vi "OnePointSub.vi"(3 "cluster":T1) -> (0 "TextArray":string[](array[string]), 1 "Array":dbl[](array[numeric]))   [LabVIEW 2017]
panel:
  out "Numeric 3":i32
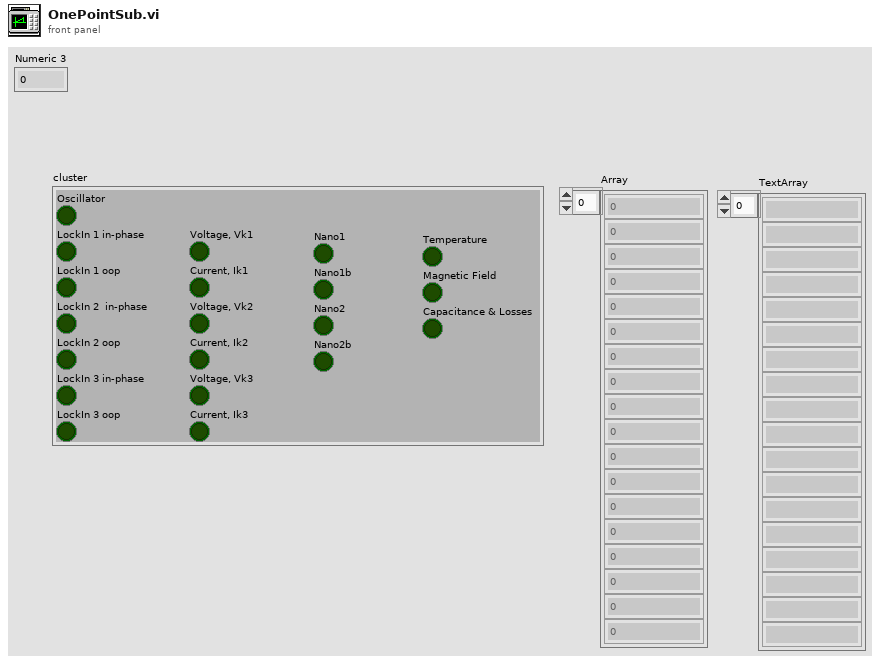
[diagram p1: front panel]
types:
  T1 = cluster{"Oscillator":bool, "LockIn 1 in-phase":bool, "LockIn 1 oop ":bool, "LockIn 2  in-phase":bool, "LockIn 2 oop":bool, "LockIn 3 in-phase":bool, "LockIn 3 oop":bool, "Voltage, Vk1":bool, "Current, Ik1":bool, "Voltage, Vk2":bool, "Current, Ik2":bool, "Voltage, Vk3":bool, "Current, Ik3":bool, "Nano1":bool, "Nano1b":bool, "Nano2":bool, "Nano2b":bool, "Temperature":bool, "Magnetic Field":bool, "Capacitance & Losses":bool}
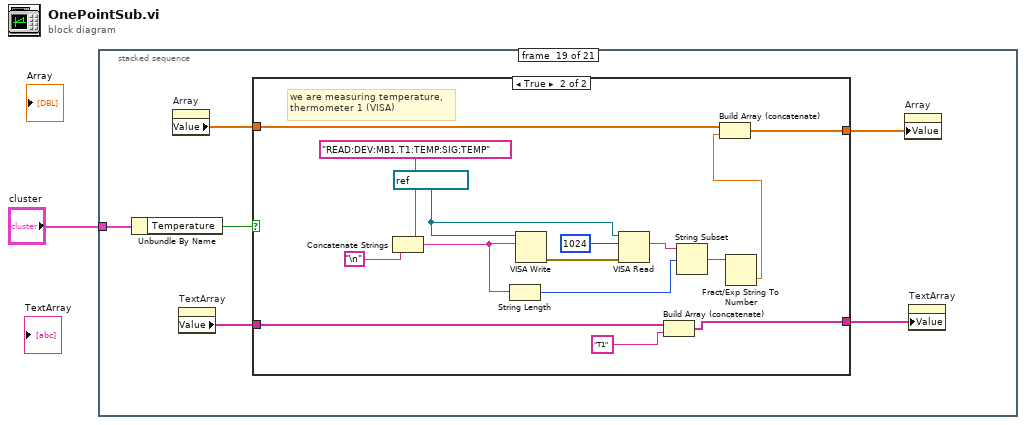
[diagram p0: block diagram]
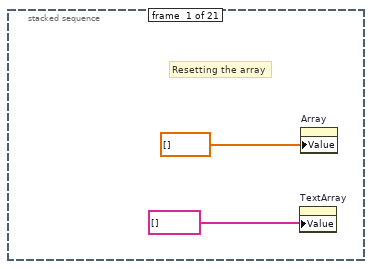
[diagram p2: hidden frame]
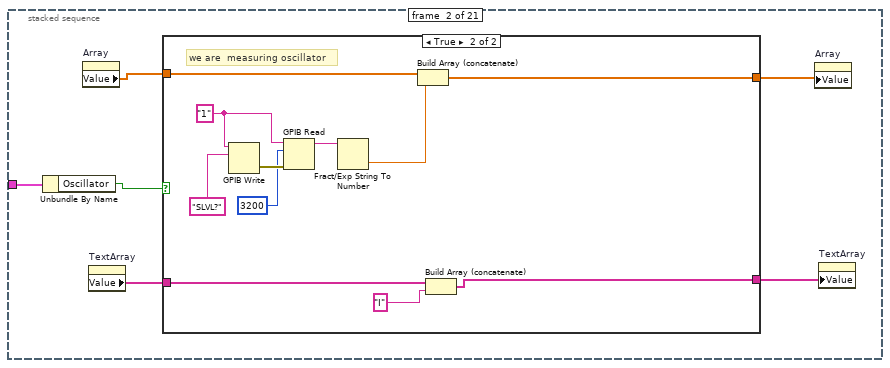
[diagram p3: hidden frame]
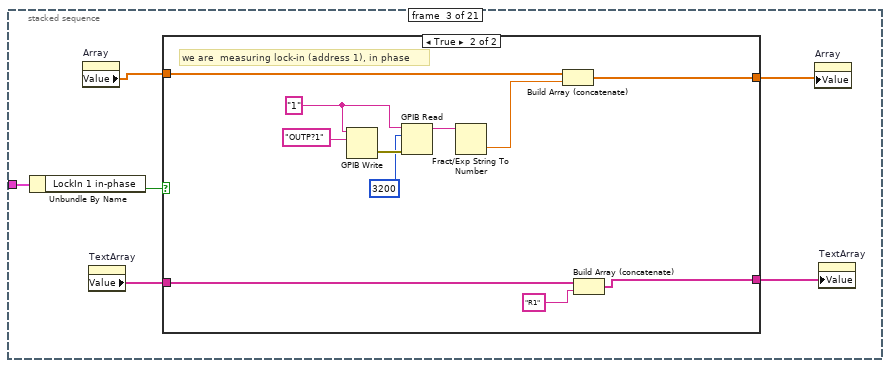
[diagram p5: hidden frame]
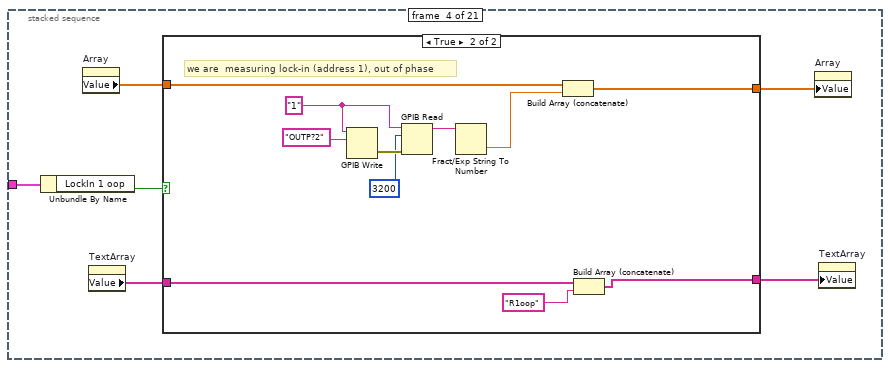
[diagram p7: hidden frame]
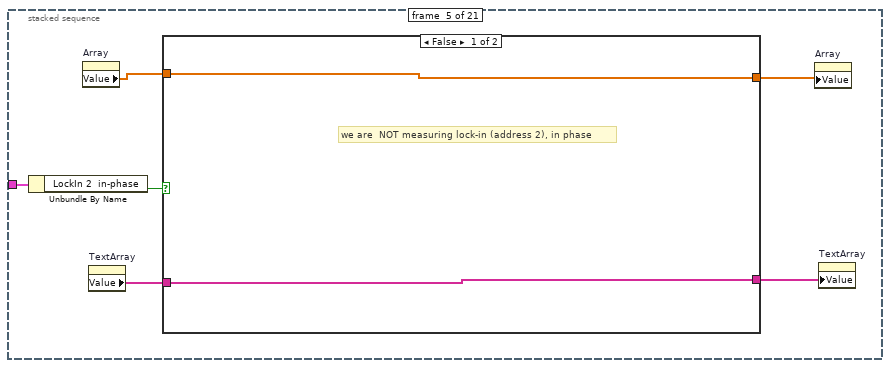
[diagram p9: hidden frame]
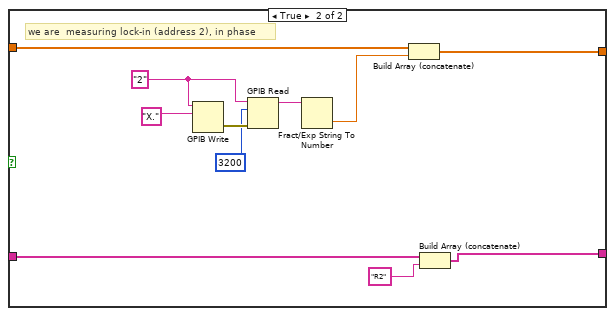
[diagram p10: hidden frame]
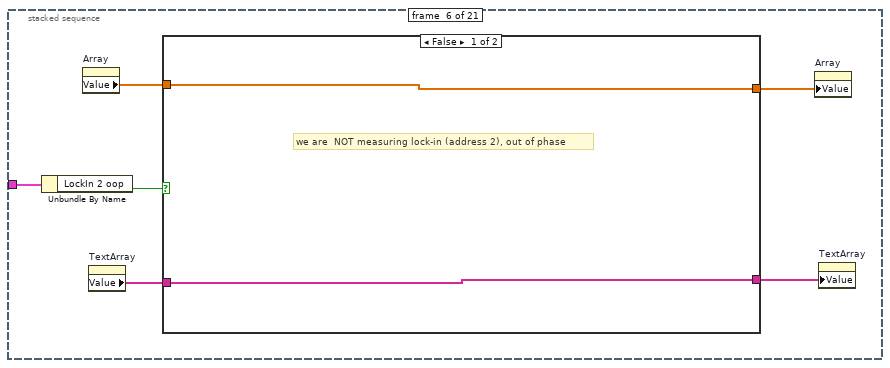
[diagram p11: hidden frame]
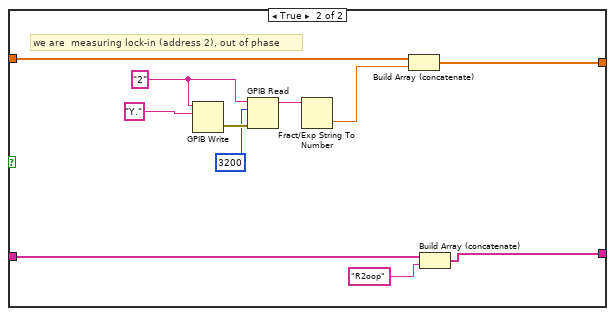
[diagram p12: hidden frame]
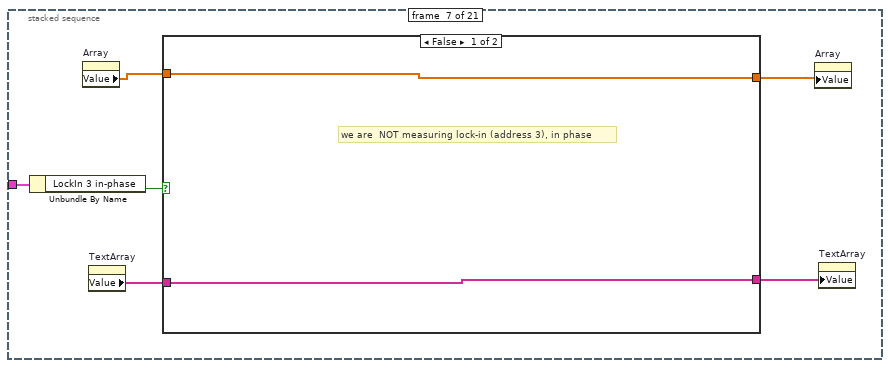
[diagram p13: hidden frame]
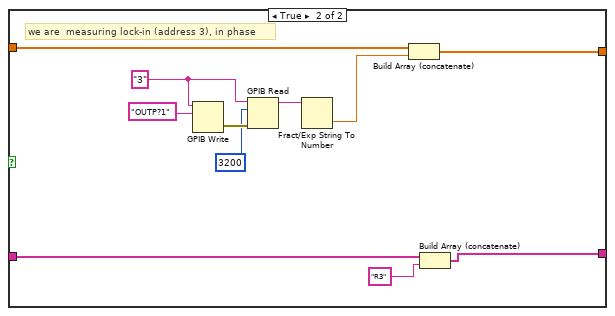
[diagram p14: hidden frame]
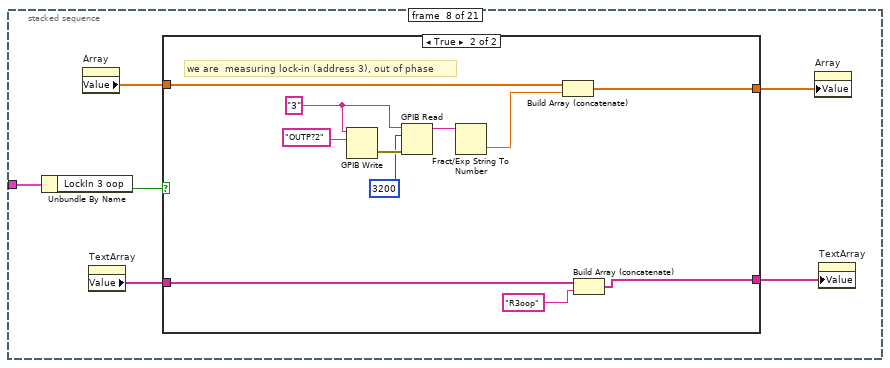
[diagram p15: hidden frame]
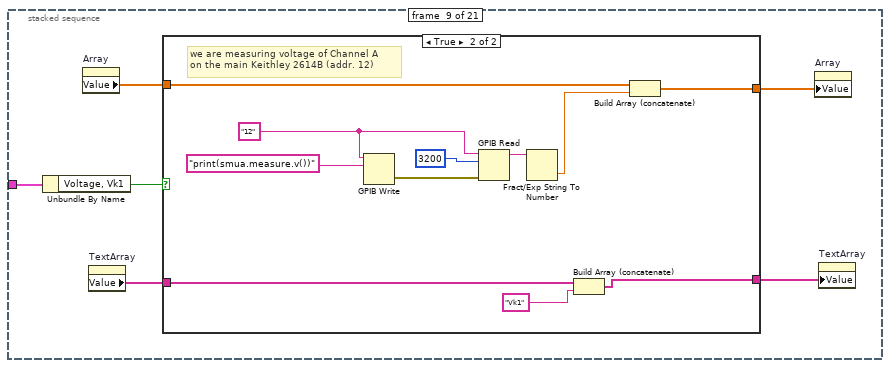
[diagram p17: hidden frame]
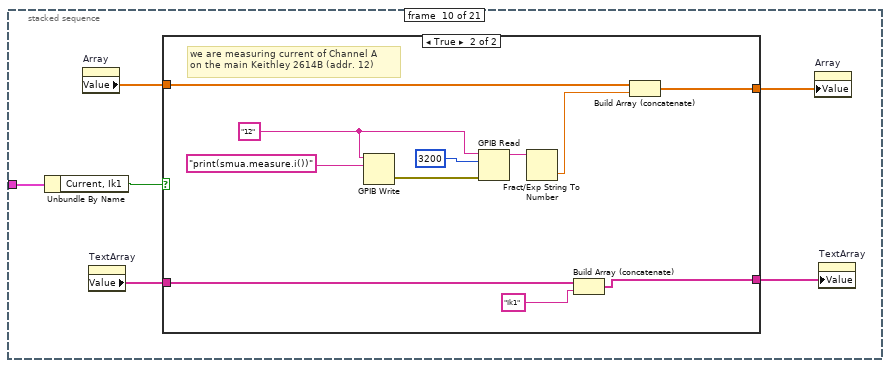
[diagram p19: hidden frame]
diagram:
  n1 = stacked-sequence {
    tunnel: "cluster" -> [_ w9 w28 w47 w66 w85 w104 w123 w142 w161 w180 w199 w218 w237 w256 w275 w298 w317 w340 w363 w386]
    frame #0 {
      # "Resetting the array"
      n2 = property on="TextArray" class="Arr (strict)"("Value"=string[] []) -> ()  [unwired: 2 in, 2 out]
      n3 = property on="Array" class="Arr (strict)"("Value"=dbl[] []) -> ()  [unwired: 2 in, 2 out]
    }
    frame #1 {
      n4 = Unbundle By Name(w9) -> ("Oscillator"=w6:bool)
      n5 = property on="Array" class="Arr (strict)"() -> ("Value"=w8:dbl[])  [unwired: 2 in, 2 out]
      n6 = property on="TextArray" class="Arr (strict)"() -> ("Value"=w5:string[])  [unwired: 2 in, 2 out]
      n7 = case shown="True" w6 {
        tunnel: w8 -> [w11 w22]
        tunnel: [w11 w21] -> w7
        tunnel: w5 -> [w10 w14]
        tunnel: [w10 w13] -> w4
        frame False {
          # "we are not measuring oscillator from\nlock-in (address 1)"
        }
        frame True {
          w18 = "1"
          # "we are  measuring oscillator"
          n8 = GPIB Write(0:w18, 1:"SLVL?") -> (6:w19:errorcluster)  [unwired: 3 in, 1 out]
          n9 = GPIB Read(0:w18, 1:3200, 3:w19) -> (5:w16:string)  [unwired: 2 in, 2 out]
          n10 = Fract/Exp String To Number(string=w16) -> (number=w15:dbl)  [unwired: 3 in, 1 out]
          n11 = Build Array (concatenate)(w22, w15) -> (w21:dbl[])
          n12 = Build Array (concatenate)(w14, "I") -> (w13:string[])
        }
      }
      n13 = property on="Array" class="Arr (strict)"("Value"=w7) -> ()  [unwired: 2 in, 2 out]
      n14 = property on="TextArray" class="Arr (strict)"("Value"=w4) -> ()  [unwired: 2 in, 2 out]
    }
    frame #2 {
      n15 = Unbundle By Name(w28) -> ("LockIn 1 in-phase"=w25:bool)
      n16 = property on="Array" class="Arr (strict)"() -> ("Value"=w27:dbl[])  [unwired: 2 in, 2 out]
      n17 = property on="TextArray" class="Arr (strict)"() -> ("Value"=w24:string[])  [unwired: 2 in, 2 out]
      n18 = case shown="True" w25 {
        tunnel: w27 -> [w30 w41]
        tunnel: [w30 w40] -> w26
        tunnel: w24 -> [w29 w39]
        tunnel: [w29 w38] -> w23
        frame False {
          # "we are  NOT measuring lock-in (address 1), in phase"
        }
        frame True {
          w35 = "1"
          # "we are  measuring lock-in (address 1), in phase"
          n19 = GPIB Write(0:w35, 1:"OUTP?1") -> (6:w36:errorcluster)  [unwired: 3 in, 1 out]
          n20 = GPIB Read(0:w35, 1:3200, 3:w36) -> (5:w33:string)  [unwired: 2 in, 2 out]
          n21 = Fract/Exp String To Number(string=w33) -> (number=w31:dbl)  [unwired: 3 in, 1 out]
          n22 = Build Array (concatenate)(w41, w31) -> (w40:dbl[])
          n23 = Build Array (concatenate)(w39, "R1") -> (w38:string[])
        }
      }
      n24 = property on="Array" class="Arr (strict)"("Value"=w26) -> ()  [unwired: 2 in, 2 out]
      n25 = property on="TextArray" class="Arr (strict)"("Value"=w23) -> ()  [unwired: 2 in, 2 out]
    }
    frame #3 {
      n26 = Unbundle By Name(w47) -> ("LockIn 1 oop"=w44:bool)
      n27 = property on="Array" class="Arr (strict)"() -> ("Value"=w46:dbl[])  [unwired: 2 in, 2 out]
      n28 = property on="TextArray" class="Arr (strict)"() -> ("Value"=w43:string[])  [unwired: 2 in, 2 out]
      n29 = case shown="True" w44 {
        tunnel: w46 -> [w49 w60]
        tunnel: [w49 w59] -> w45
        tunnel: w43 -> [w48 w58]
        tunnel: [w48 w57] -> w42
        frame False {
          # "we are  NOT measuring lock-in (address 1), out of phase"
        }
        frame True {
          w54 = "1"
          # "we are  measuring lock-in (address 1), out of phase"
          n30 = GPIB Write(0:w54, 1:"OUTP?2") -> (6:w55:errorcluster)  [unwired: 3 in, 1 out]
          n31 = GPIB Read(0:w54, 1:3200, 3:w55) -> (5:w52:string)  [unwired: 2 in, 2 out]
          n32 = Fract/Exp String To Number(string=w52) -> (number=w50:dbl)  [unwired: 3 in, 1 out]
          n33 = Build Array (concatenate)(w60, w50) -> (w59:dbl[])
          n34 = Build Array (concatenate)(w58, "R1oop") -> (w57:string[])
        }
      }
      n35 = property on="Array" class="Arr (strict)"("Value"=w45) -> ()  [unwired: 2 in, 2 out]
      n36 = property on="TextArray" class="Arr (strict)"("Value"=w42) -> ()  [unwired: 2 in, 2 out]
    }
    frame #4 {
      n37 = Unbundle By Name(w66) -> ("LockIn 2  in-phase"=w63:bool)
      n38 = property on="Array" class="Arr (strict)"() -> ("Value"=w65:dbl[])  [unwired: 2 in, 2 out]
      n39 = property on="TextArray" class="Arr (strict)"() -> ("Value"=w62:string[])  [unwired: 2 in, 2 out]
      n40 = case shown="False" w63 {
        tunnel: w65 -> [w68 w79]
        tunnel: [w68 w78] -> w64
        tunnel: w62 -> [w67 w77]
        tunnel: [w67 w76] -> w61
        frame False {
          # "we are  NOT measuring lock-in (address 2), in phase"
        }
        frame True {
          w73 = "2"
          # "we are  measuring lock-in (address 2), in phase"
          n41 = GPIB Write(0:w73, 1:"X.") -> (6:w74:errorcluster)  [unwired: 3 in, 1 out]
          n42 = GPIB Read(0:w73, 1:3200, 3:w74) -> (5:w71:string)  [unwired: 2 in, 2 out]
          n43 = Fract/Exp String To Number(string=w71) -> (number=w70:dbl)  [unwired: 3 in, 1 out]
          n44 = Build Array (concatenate)(w79, w70) -> (w78:dbl[])
          n45 = Build Array (concatenate)(w77, "R2") -> (w76:string[])
        }
      }
      n46 = property on="Array" class="Arr (strict)"("Value"=w64) -> ()  [unwired: 2 in, 2 out]
      n47 = property on="TextArray" class="Arr (strict)"("Value"=w61) -> ()  [unwired: 2 in, 2 out]
    }
    frame #5 {
      n48 = Unbundle By Name(w85) -> ("LockIn 2 oop"=w82:bool)
      n49 = property on="Array" class="Arr (strict)"() -> ("Value"=w84:dbl[])  [unwired: 2 in, 2 out]
      n50 = property on="TextArray" class="Arr (strict)"() -> ("Value"=w81:string[])  [unwired: 2 in, 2 out]
      n51 = case shown="False" w82 {
        tunnel: w84 -> [w87 w98]
        tunnel: [w87 w97] -> w83
        tunnel: w81 -> [w86 w96]
        tunnel: [w86 w95] -> w80
        frame False {
          # "we are  NOT measuring lock-in (address 2), out of phase"
        }
        frame True {
          w92 = "2"
          # "we are  measuring lock-in (address 2), out of phase"
          n52 = GPIB Write(0:w92, 1:"Y.") -> (6:w93:errorcluster)  [unwired: 3 in, 1 out]
          n53 = GPIB Read(0:w92, 1:3200, 3:w93) -> (5:w90:string)  [unwired: 2 in, 2 out]
          n54 = Fract/Exp String To Number(string=w90) -> (number=w88:dbl)  [unwired: 3 in, 1 out]
          n55 = Build Array (concatenate)(w98, w88) -> (w97:dbl[])
          n56 = Build Array (concatenate)(w96, "R2oop") -> (w95:string[])
        }
      }
      n57 = property on="Array" class="Arr (strict)"("Value"=w83) -> ()  [unwired: 2 in, 2 out]
      n58 = property on="TextArray" class="Arr (strict)"("Value"=w80) -> ()  [unwired: 2 in, 2 out]
    }
    frame #6 {
      n59 = Unbundle By Name(w104) -> ("LockIn 3 in-phase"=w101:bool)
      n60 = property on="Array" class="Arr (strict)"() -> ("Value"=w103:dbl[])  [unwired: 2 in, 2 out]
      n61 = property on="TextArray" class="Arr (strict)"() -> ("Value"=w100:string[])  [unwired: 2 in, 2 out]
      n62 = case shown="False" w101 {
        tunnel: w103 -> [w106 w117]
        tunnel: [w106 w116] -> w102
        tunnel: w100 -> [w105 w115]
        tunnel: [w105 w114] -> w99
        frame False {
          # "we are  NOT measuring lock-in (address 3), in phase"
        }
        frame True {
          w111 = "3"
          # "we are  measuring lock-in (address 3), in phase"
          n63 = GPIB Write(0:w111, 1:"OUTP?1") -> (6:w112:errorcluster)  [unwired: 3 in, 1 out]
          n64 = GPIB Read(0:w111, 1:3200, 3:w112) -> (5:w109:string)  [unwired: 2 in, 2 out]
          n65 = Fract/Exp String To Number(string=w109) -> (number=w107:dbl)  [unwired: 3 in, 1 out]
          n66 = Build Array (concatenate)(w117, w107) -> (w116:dbl[])
          n67 = Build Array (concatenate)(w115, "R3") -> (w114:string[])
        }
      }
      n68 = property on="Array" class="Arr (strict)"("Value"=w102) -> ()  [unwired: 2 in, 2 out]
      n69 = property on="TextArray" class="Arr (strict)"("Value"=w99) -> ()  [unwired: 2 in, 2 out]
    }
    frame #7 {
      n70 = Unbundle By Name(w123) -> ("LockIn 3 oop"=w120:bool)
      n71 = property on="Array" class="Arr (strict)"() -> ("Value"=w122:dbl[])  [unwired: 2 in, 2 out]
      n72 = property on="TextArray" class="Arr (strict)"() -> ("Value"=w119:string[])  [unwired: 2 in, 2 out]
      n73 = case shown="True" w120 {
        tunnel: w122 -> [w125 w136]
        tunnel: [w125 w135] -> w121
        tunnel: w119 -> [w124 w134]
        tunnel: [w124 w133] -> w118
        frame False {
          # "we are  NOT measuring lock-in (address 3), out of phase"
        }
        frame True {
          w130 = "3"
          # "we are  measuring lock-in (address 3), out of phase"
          n74 = GPIB Write(0:w130, 1:"OUTP?2") -> (6:w131:errorcluster)  [unwired: 3 in, 1 out]
          n75 = GPIB Read(0:w130, 1:3200, 3:w131) -> (5:w128:string)  [unwired: 2 in, 2 out]
          n76 = Fract/Exp String To Number(string=w128) -> (number=w126:dbl)  [unwired: 3 in, 1 out]
          n77 = Build Array (concatenate)(w136, w126) -> (w135:dbl[])
          n78 = Build Array (concatenate)(w134, "R3oop") -> (w133:string[])
        }
      }
      n79 = property on="Array" class="Arr (strict)"("Value"=w121) -> ()  [unwired: 2 in, 2 out]
      n80 = property on="TextArray" class="Arr (strict)"("Value"=w118) -> ()  [unwired: 2 in, 2 out]
    }
    frame #8 {
      n81 = Unbundle By Name(w142) -> ("Voltage, Vk1"=w139:bool)
      n82 = property on="Array" class="Arr (strict)"() -> ("Value"=w141:dbl[])  [unwired: 2 in, 2 out]
      n83 = property on="TextArray" class="Arr (strict)"() -> ("Value"=w138:string[])  [unwired: 2 in, 2 out]
      n84 = case shown="True" w139 {
        tunnel: w141 -> [w144 w155]
        tunnel: [w144 w154] -> w140
        tunnel: w138 -> [w143 w153]
        tunnel: [w143 w152] -> w137
        frame False {
          # "we are NOT measuring voltage of Channel A \non the main Keithley 2614B (addr. 12)"
        }
        frame True {
          w149 = "12"
          # "we are measuring voltage of Channel A \non the main Keithley 2614B (addr. 12)"
          n85 = GPIB Write(0:w149, 1:"print(smua.measure.v())") -> (6:w150:errorcluster)  [unwired: 3 in, 1 out]
          n86 = GPIB Read(0:w149, 1:3200, 3:w150) -> (5:w146:string)  [unwired: 2 in, 2 out]
          n87 = Fract/Exp String To Number(string=w146) -> (number=w145:dbl)  [unwired: 3 in, 1 out]
          n88 = Build Array (concatenate)(w153, "Vk1") -> (w152:string[])
          n89 = Build Array (concatenate)(w155, w145) -> (w154:dbl[])
        }
      }
      n90 = property on="Array" class="Arr (strict)"("Value"=w140) -> ()  [unwired: 2 in, 2 out]
      n91 = property on="TextArray" class="Arr (strict)"("Value"=w137) -> ()  [unwired: 2 in, 2 out]
    }
    frame #9 {
      n92 = Unbundle By Name(w161) -> ("Current, Ik1"=w158:bool)
      n93 = property on="Array" class="Arr (strict)"() -> ("Value"=w160:dbl[])  [unwired: 2 in, 2 out]
      n94 = property on="TextArray" class="Arr (strict)"() -> ("Value"=w157:string[])  [unwired: 2 in, 2 out]
      n95 = case shown="True" w158 {
        tunnel: w160 -> [w163 w174]
        tunnel: [w163 w173] -> w159
        tunnel: w157 -> [w162 w172]
        tunnel: [w162 w171] -> w156
        frame False {
          # "we are NOT measuring current of Channel A \non the main Keithley 2614B (addr. 12)"
        }
        frame True {
          w168 = "12"
          # "we are measuring current of Channel A \non the main Keithley 2614B (addr. 12)"
          n96 = GPIB Write(0:w168, 1:"print(smua.measure.i())") -> (6:w169:errorcluster)  [unwired: 3 in, 1 out]
          n97 = GPIB Read(0:w168, 1:3200, 3:w169) -> (5:w165:string)  [unwired: 2 in, 2 out]
          n98 = Fract/Exp String To Number(string=w165) -> (number=w164:dbl)  [unwired: 3 in, 1 out]
          n99 = Build Array (concatenate)(w172, "Ik1") -> (w171:string[])
          n100 = Build Array (concatenate)(w174, w164) -> (w173:dbl[])
        }
      }
      n101 = property on="Array" class="Arr (strict)"("Value"=w159) -> ()  [unwired: 2 in, 2 out]
      n102 = property on="TextArray" class="Arr (strict)"("Value"=w156) -> ()  [unwired: 2 in, 2 out]
    }
    frame #10 {
      n103 = Unbundle By Name(w180) -> ("Voltage, Vk2"=w177:bool)
      n104 = property on="Array" class="Arr (strict)"() -> ("Value"=w179:dbl[])  [unwired: 2 in, 2 out]
      n105 = property on="TextArray" class="Arr (strict)"() -> ("Value"=w176:string[])  [unwired: 2 in, 2 out]
      n106 = case shown="True" w177 {
        tunnel: w179 -> [w182 w193]
        tunnel: [w182 w192] -> w178
        tunnel: w176 -> [w181 w191]
        tunnel: [w181 w190] -> w175
        frame False {
          # "we are NOT measuring voltage of Channel B \non the main Keithley 2614B (addr. 12)"
        }
        frame True {
          w187 = "12"
          # "we are measuring voltage of Channel B \non the main Keithley 2614B (addr. 12)"
          n107 = GPIB Write(0:w187, 1:"print(smub.measure.v())") -> (6:w188:errorcluster)  [unwired: 3 in, 1 out]
          n108 = GPIB Read(0:w187, 1:3200, 3:w188) -> (5:w184:string)  [unwired: 2 in, 2 out]
          n109 = Fract/Exp String To Number(string=w184) -> (number=w183:dbl)  [unwired: 3 in, 1 out]
          n110 = Build Array (concatenate)(w191, "Vk2") -> (w190:string[])
          n111 = Build Array (concatenate)(w193, w183) -> (w192:dbl[])
        }
      }
      n112 = property on="Array" class="Arr (strict)"("Value"=w178) -> ()  [unwired: 2 in, 2 out]
      n113 = property on="TextArray" class="Arr (strict)"("Value"=w175) -> ()  [unwired: 2 in, 2 out]
    }
    frame #11 {
      n114 = Unbundle By Name(w199) -> ("Current, Ik2"=w196:bool)
      n115 = property on="Array" class="Arr (strict)"() -> ("Value"=w198:dbl[])  [unwired: 2 in, 2 out]
      n116 = property on="TextArray" class="Arr (strict)"() -> ("Value"=w195:string[])  [unwired: 2 in, 2 out]
      n117 = case shown="True" w196 {
        tunnel: w198 -> [w201 w212]
        tunnel: [w201 w211] -> w197
        tunnel: w195 -> [w200 w210]
        tunnel: [w200 w209] -> w194
        frame False {
          # "we are NOT measuring current of Channel B \non the main Keithley 2614B (addr. 12)"
        }
        frame True {
          w206 = "12"
          # "we are measuring current of Channel B \non the main Keithley 2614B (addr. 12)"
          n118 = GPIB Write(0:w206, 1:"print(smub.measure.i())") -> (6:w207:errorcluster)  [unwired: 3 in, 1 out]
          n119 = GPIB Read(0:w206, 1:3200, 3:w207) -> (5:w203:string)  [unwired: 2 in, 2 out]
          n120 = Fract/Exp String To Number(string=w203) -> (number=w202:dbl)  [unwired: 3 in, 1 out]
          n121 = Build Array (concatenate)(w210, "Ik2") -> (w209:string[])
          n122 = Build Array (concatenate)(w212, w202) -> (w211:dbl[])
        }
      }
      n123 = property on="Array" class="Arr (strict)"("Value"=w197) -> ()  [unwired: 2 in, 2 out]
      n124 = property on="TextArray" class="Arr (strict)"("Value"=w194) -> ()  [unwired: 2 in, 2 out]
    }
    frame #12 {
      n125 = Unbundle By Name(w218) -> ("Voltage, Vk3"=w215:bool)
      n126 = property on="Array" class="Arr (strict)"() -> ("Value"=w217:dbl[])  [unwired: 2 in, 2 out]
      n127 = property on="TextArray" class="Arr (strict)"() -> ("Value"=w214:string[])  [unwired: 2 in, 2 out]
      n128 = case shown="True" w215 {
        tunnel: w217 -> [w220 w231]
        tunnel: [w220 w230] -> w216
        tunnel: w214 -> [w219 w229]
        tunnel: [w219 w228] -> w213
        frame False {
          # "we are NOT measuring voltage of Channel B \non the main Keithley 2614B (addr. 12)"
        }
        frame True {
          w225 = "13"
          # "RESERVED"
          # "we are measuring voltage of Channel A \non the main Keithley 2614B (addr. 13)"
          n129 = GPIB Write(0:w225, 1:"print(smub.measure.v())") -> (6:w226:errorcluster)  [unwired: 3 in, 1 out]
          n130 = GPIB Read(0:w225, 1:3200, 3:w226) -> (5:w222:string)  [unwired: 2 in, 2 out]
          n131 = Fract/Exp String To Number(string=w222) -> (number=w221:dbl)  [unwired: 3 in, 1 out]
          n132 = Build Array (concatenate)(w229, "Vk3") -> (w228:string[])
          n133 = Build Array (concatenate)(w231, w221) -> (w230:dbl[])
        }
      }
      n134 = property on="Array" class="Arr (strict)"("Value"=w216) -> ()  [unwired: 2 in, 2 out]
      n135 = property on="TextArray" class="Arr (strict)"("Value"=w213) -> ()  [unwired: 2 in, 2 out]
    }
    frame #13 {
      n136 = Unbundle By Name(w237) -> ("Current, Ik3"=w234:bool)
      n137 = property on="Array" class="Arr (strict)"() -> ("Value"=w236:dbl[])  [unwired: 2 in, 2 out]
      n138 = property on="TextArray" class="Arr (strict)"() -> ("Value"=w233:string[])  [unwired: 2 in, 2 out]
      n139 = case shown="True" w234 {
        tunnel: w236 -> [w239 w250]
        tunnel: [w239 w249] -> w235
        tunnel: w233 -> [w238 w248]
        tunnel: [w238 w247] -> w232
        frame False {
          # "we are NOT measuring current of Channel B \non the main Keithley 2614B (addr. 12)"
        }
        frame True {
          w244 = "13"
          # "RESERVED"
          # "we are measuring current of Channel B \non the main Keithley 2614B (addr. 12)"
          n140 = GPIB Write(0:w244, 1:"print(smua.measure.i())") -> (6:w245:errorcluster)  [unwired: 3 in, 1 out]
          n141 = GPIB Read(0:w244, 1:3200, 3:w245) -> (5:w241:string)  [unwired: 2 in, 2 out]
          n142 = Fract/Exp String To Number(string=w241) -> (number=w240:dbl)  [unwired: 3 in, 1 out]
          n143 = Build Array (concatenate)(w248, "Ik3") -> (w247:string[])
          n144 = Build Array (concatenate)(w250, w240) -> (w249:dbl[])
        }
      }
      n145 = property on="Array" class="Arr (strict)"("Value"=w235) -> ()  [unwired: 2 in, 2 out]
      n146 = property on="TextArray" class="Arr (strict)"("Value"=w232) -> ()  [unwired: 2 in, 2 out]
    }
    frame #14 {
      n147 = Unbundle By Name(w256) -> ("Nano1"=w253:bool)
      n148 = property on="Array" class="Arr (strict)"() -> ("Value"=w255:dbl[])  [unwired: 2 in, 2 out]
      n149 = property on="TextArray" class="Arr (strict)"() -> ("Value"=w252:string[])  [unwired: 2 in, 2 out]
      n150 = case shown="True" w253 {
        tunnel: w255 -> [w258 w269]
        tunnel: [w258 w268] -> w254
        tunnel: w252 -> [w257 w267]
        tunnel: [w257 w266] -> w251
        frame False {
          # "we are NOT measuring current of Channel B \non the main Keithley 2614B (addr. 12)"
        }
        frame True {
          w263 = "15"
          # "we are measuring 1st channel\non Keithley 2182 (addr. 15)"
          n151 = GPIB Write(0:w263, 1:":SENSe:DATA:FRES?") -> (6:w264:errorcluster)  [unwired: 3 in, 1 out]
          n152 = GPIB Read(0:w263, 1:200, 3:w264) -> (5:w260:string)  [unwired: 2 in, 2 out]
          n153 = Fract/Exp String To Number(string=w260) -> (number=w259:dbl)  [unwired: 3 in, 1 out]
          n154 = Build Array (concatenate)(w267, "Vnano1") -> (w266:string[])
          n155 = Build Array (concatenate)(w269, w259) -> (w268:dbl[])
        }
      }
      n156 = property on="Array" class="Arr (strict)"("Value"=w254) -> ()  [unwired: 2 in, 2 out]
      n157 = property on="TextArray" class="Arr (strict)"("Value"=w251) -> ()  [unwired: 2 in, 2 out]
    }
    frame #15 {
      n158 = Unbundle By Name(w275) -> ("Nano1b"=w272:bool)
      n159 = property on="Array" class="Arr (strict)"() -> ("Value"=w274:dbl[])  [unwired: 2 in, 2 out]
      n160 = property on="TextArray" class="Arr (strict)"() -> ("Value"=w271:string[])  [unwired: 2 in, 2 out]
      n161 = case shown="True" w272 {
        tunnel: w274 -> [w277 w292]
        tunnel: [w277 w291] -> w273
        tunnel: w271 -> [w276 w290]
        tunnel: [w276 w289] -> w270
        frame False {
          # "we are NOT measuring current of Channel B \non the main Keithley 2614B (addr. 12)"
        }
        frame True {
          w281 = "15"
          # "switching to channel 2 and then\nback to channel 1"
          # "we are measuring 2nd channel\non Keithley 2182 (addr. 15)"
          n162 = GPIB Write(0:w281, 1:":SENSe:CHAN 2") -> (6:w282:errorcluster)  [unwired: 3 in, 1 out]
          n163 = GPIB Write(0:w281, 1:":SENSe:DATA:FRES?", 3:w282) -> (6:w287:errorcluster)  [unwired: 2 in, 1 out]
          n164 = GPIB Read(0:w281, 1:200, 3:w287) -> (5:w284:string, 7:w280:errorcluster)  [unwired: 2 in, 1 out]
          n165 = GPIB Write(0:w281, 1:":SENSe:CHAN 1", 3:w280) -> ()  [unwired: 2 in, 2 out]
          n166 = Build Array (concatenate)(w290, "Vnano1b") -> (w289:string[])
          n167 = Fract/Exp String To Number(string=w284) -> (number=w278:dbl)  [unwired: 3 in, 1 out]
          n168 = Build Array (concatenate)(w292, w278) -> (w291:dbl[])
        }
      }
      n169 = property on="Array" class="Arr (strict)"("Value"=w273) -> ()  [unwired: 2 in, 2 out]
      n170 = property on="TextArray" class="Arr (strict)"("Value"=w270) -> ()  [unwired: 2 in, 2 out]
    }
    frame #16 {
      n171 = Unbundle By Name(w298) -> ("Nano2"=w295:bool)
      n172 = property on="Array" class="Arr (strict)"() -> ("Value"=w297:dbl[])  [unwired: 2 in, 2 out]
      n173 = property on="TextArray" class="Arr (strict)"() -> ("Value"=w294:string[])  [unwired: 2 in, 2 out]
      n174 = case shown="True" w295 {
        tunnel: w297 -> [w300 w311]
        tunnel: [w300 w310] -> w296
        tunnel: w294 -> [w299 w309]
        tunnel: [w299 w308] -> w293
        frame False {
          # "we are NOT measuring current of Channel B \non the main Keithley 2614B (addr. 12)"
        }
        frame True {
          w305 = "16"
          # "RESERVED"
          # "we are measuring 1st channel\non Keithley 2182 (addr. 16)"
          n175 = GPIB Write(0:w305, 1:":SENSe:DATA:FRES?") -> (6:w306:errorcluster)  [unwired: 3 in, 1 out]
          n176 = GPIB Read(0:w305, 1:200, 3:w306) -> (5:w302:string)  [unwired: 2 in, 2 out]
          n177 = Fract/Exp String To Number(string=w302) -> (number=w301:dbl)  [unwired: 3 in, 1 out]
          n178 = Build Array (concatenate)(w309, "Vnano2") -> (w308:string[])
          n179 = Build Array (concatenate)(w311, w301) -> (w310:dbl[])
        }
      }
      n180 = property on="Array" class="Arr (strict)"("Value"=w296) -> ()  [unwired: 2 in, 2 out]
      n181 = property on="TextArray" class="Arr (strict)"("Value"=w293) -> ()  [unwired: 2 in, 2 out]
    }
    frame #17 {
      n182 = Unbundle By Name(w317) -> ("Nano2b"=w314:bool)
      n183 = property on="Array" class="Arr (strict)"() -> ("Value"=w316:dbl[])  [unwired: 2 in, 2 out]
      n184 = property on="TextArray" class="Arr (strict)"() -> ("Value"=w313:string[])  [unwired: 2 in, 2 out]
      n185 = case shown="True" w314 {
        tunnel: w316 -> [w319 w334]
        tunnel: [w319 w333] -> w315
        tunnel: w313 -> [w318 w332]
        tunnel: [w318 w331] -> w312
        frame False {
          # "we are NOT measuring current of Channel B \non the main Keithley 2614B (addr. 12)"
        }
        frame True {
          w323 = "16"
          # "switching to channel 2 and then\nback to channel 1"
          # "we are measuring 2nd channel\non Keithley 2182 (addr. 16)"
          n186 = GPIB Write(0:w323, 1:":SENSe:CHAN 2") -> (6:w324:errorcluster)  [unwired: 3 in, 1 out]
          n187 = GPIB Write(0:w323, 1:":SENSe:DATA:FRES?", 3:w324) -> (6:w329:errorcluster)  [unwired: 2 in, 1 out]
          n188 = GPIB Read(0:w323, 1:200, 3:w329) -> (5:w326:string, 7:w322:errorcluster)  [unwired: 2 in, 1 out]
          n189 = GPIB Write(0:w323, 1:":SENSe:CHAN 1", 3:w322) -> ()  [unwired: 2 in, 2 out]
          n190 = Build Array (concatenate)(w332, "Vnano2b") -> (w331:string[])
          n191 = Fract/Exp String To Number(string=w326) -> (number=w320:dbl)  [unwired: 3 in, 1 out]
          n192 = Build Array (concatenate)(w334, w320) -> (w333:dbl[])
        }
      }
      n193 = property on="Array" class="Arr (strict)"("Value"=w315) -> ()  [unwired: 2 in, 2 out]
      n194 = property on="TextArray" class="Arr (strict)"("Value"=w312) -> ()  [unwired: 2 in, 2 out]
    }
    frame #18 {
      n195 = Unbundle By Name(w340) -> ("Temperature"=w337:bool)
      n196 = property on="Array" class="Arr (strict)"() -> ("Value"=w339:dbl[])  [unwired: 2 in, 2 out]
      n197 = property on="TextArray" class="Arr (strict)"() -> ("Value"=w336:string[])  [unwired: 2 in, 2 out]
      n198 = case shown="True" w337 {
        tunnel: w339 -> [w342 w357]
        tunnel: [w342 w356] -> w338
        tunnel: w336 -> [w341 w355]
        tunnel: [w341 w354] -> w335
        frame False {
          # "we are NOT measuring temperature"
        }
        frame True {
          w347 = refnum<visa-resource-name> "itcetherT" ("VISA resource name")
          # "we are measuring temperature,\nthermometer 1 (VISA)"
          n199 = Concatenate Strings("READ:DEV:MB1.T1:TEMP:SIG:TEMP" ("string"), "\n") -> (w346:string)
          n200 = String Length(string=w346) -> (length=w344:i32)
          n201 = VISA Write(VISA resource name=w347, write buffer=w346) -> (error out=w352:errorcluster)  [unwired: 1 in, 2 out]
          n202 = VISA Read(VISA resource name=w347, byte count=1024, error in (no error)=w352) -> (read buffer=w350:string)  [unwired: 3 out]
          n203 = Build Array (concatenate)(w355, "T1") -> (w354:string[])
          n204 = String Subset(string=w350, offset (0)=w344) -> (substring=w349:string)  [unwired: 1 in]
          n205 = Fract/Exp String To Number(string=w349) -> (number=w343:dbl)  [unwired: 3 in, 1 out]
          n206 = Build Array (concatenate)(w357, w343) -> (w356:dbl[])
        }
      }
      n207 = property on="Array" class="Arr (strict)"("Value"=w338) -> ()  [unwired: 2 in, 2 out]
      n208 = property on="TextArray" class="Arr (strict)"("Value"=w335) -> ()  [unwired: 2 in, 2 out]
    }
    frame #19 {
      n209 = Unbundle By Name(w363) -> ("Magnetic Field"=w360:bool)
      n210 = property on="Array" class="Arr (strict)"() -> ("Value"=w362:dbl[])  [unwired: 2 in, 2 out]
      n211 = property on="TextArray" class="Arr (strict)"() -> ("Value"=w359:string[])  [unwired: 2 in, 2 out]
      n212 = case shown="True" w360 {
        tunnel: w362 -> [w365 w380]
        tunnel: [w365 w379] -> w361
        tunnel: w359 -> [w364 w378]
        tunnel: [w364 w377] -> w358
        frame False {
          # "we are NOT measuring temperature"
        }
        frame True {
          w370 = refnum<visa-resource-name> "TCPIP0::192.168.128.3::7020::SOCKET" ("VISA resource name")
          # "we are measuring magnetic field,\n(VISA)"
          n213 = Concatenate Strings("READ:DEV:GRPZ:PSU:SIG:PFLD" ("string"), "\n") -> (w369:string)
          n214 = String Length(string=w369) -> (length=w367:i32)
          n215 = VISA Write(VISA resource name=w370, write buffer=w369) -> (error out=w375:errorcluster)  [unwired: 1 in, 2 out]
          n216 = VISA Read(VISA resource name=w370, byte count=1024, error in (no error)=w375) -> (read buffer=w373:string)  [unwired: 3 out]
          n217 = Build Array (concatenate)(w378, "B") -> (w377:string[])
          n218 = String Subset(string=w373, offset (0)=w367) -> (substring=w372:string)  [unwired: 1 in]
          n219 = Fract/Exp String To Number(string=w372) -> (number=w366:dbl)  [unwired: 3 in, 1 out]
          n220 = Build Array (concatenate)(w380, w366) -> (w379:dbl[])
        }
      }
      n221 = property on="Array" class="Arr (strict)"("Value"=w361) -> ()  [unwired: 2 in, 2 out]
      n222 = property on="TextArray" class="Arr (strict)"("Value"=w358) -> ()  [unwired: 2 in, 2 out]
    }
    frame #20 {
      n223 = Unbundle By Name(w386) -> ("Capacitance & Losses"=w383:bool)
      n224 = property on="Array" class="Arr (strict)"() -> ("Value"=w385:dbl[])  [unwired: 2 in, 2 out]
      n225 = property on="TextArray" class="Arr (strict)"() -> ("Value"=w382:string[])  [unwired: 2 in, 2 out]
      n226 = case shown="True" w383 {
        tunnel: w385 -> [w388 w392]
        tunnel: [w388 w393] -> w384
        tunnel: w382 -> [w387 w389]
        tunnel: [w387 w399] -> w381
        frame False {
          # "we are NOT measuring temperature"
        }
        frame True {
          # "we are measuring capacitance and loss  (addr. 28)"
          n227 = stacked-sequence {
            tunnel: [_ _ w417] -> w394
            tunnel: [_ _ w418] -> w396
            tunnel: "28" ("data") -> [w400 w403 w412]
            frame #0 {
              n228 = GPIB Write(0:w400, 1:"SINGLE" ("data"), 2:i16 0 ("mode (0)")) -> ()  [unwired: 2 in, 2 out]
            }
            frame #1 {
              n229 = while {
                tunnel: w403 -> [w404]
                i -> [w405]
                stop <- w407 continue-if-true
                n230 = GPIB Serial Poll(0:w404) -> (2:w409:i16)  [unwired: 1 in, 2 out]
                n231 = Less?(x=w409, y=i16 128) -> (x < y?=w407:bool)
                n232 = Wait (ms)(milliseconds to wait=u32 50) -> ()  [unwired: 1 out]
                "Numeric 3" <- w405
              }
            }
            frame #2 {
              w410 = i16 2 ("mode (0)")
              n233 = GPIB Read(0:w412, 1:200 ("byte count"), 2:i16 2 ("mode (0)")) -> (5:w416:string)  [unwired: 2 in, 2 out]
              n234 = Match Pattern(string=w416, regular expression="C=") -> (after substring=w415:string)  [unwired: 1 in, 3 out]
              n235 = Match Pattern(string=w415, regular expression="PF L=") -> (after substring=w413:string)  [unwired: 1 in, 3 out]
              n236 = Search/Split String(string=w415, search string/char (-)=" ", offset (0)=w410) -> (substring before match=w420:string)  [unwired: 2 out]
              n237 = Search/Split String(string=w413, search string/char (-)=" ", offset (0)=w410) -> (substring before match=w419:string)  [unwired: 2 out]
              n238 = Fract/Exp String To Number(string=w419) -> (number=w417:dbl)  [unwired: 3 in, 1 out]
              n239 = Fract/Exp String To Number(string=w420) -> (number=w418:dbl)  [unwired: 3 in, 1 out]
            }
          }
          n240 = Build Array (concatenate)(w389, "C") -> (w390:string[])
          n241 = Build Array (concatenate)(w390, "L") -> (w399:string[])
          n242 = Build Array (concatenate)(w392, w396) -> (w395:dbl[])
          n243 = Build Array (concatenate)(w395, w394) -> (w393:dbl[])
        }
      }
      n244 = property on="Array" class="Arr (strict)"("Value"=w384) -> ()  [unwired: 2 in, 2 out]
      n245 = property on="TextArray" class="Arr (strict)"("Value"=w381) -> ()  [unwired: 2 in, 2 out]
    }
  }
